vi "check_time_method.vi"(8 "error in (no error)":errorcluster, 9 "Vrijeme od kog se broji":dbl, 10 "Proteklo vrijeme":dbl, 11 "Poslednji vremenski trenutak":dbl) -> (0 "error out":errorcluster, 1 "Status":T1, 2 "Novo proteklo vrijeme":dbl, 3 "Novi vremenski trenutak":dbl)   [LabVIEW 2023]
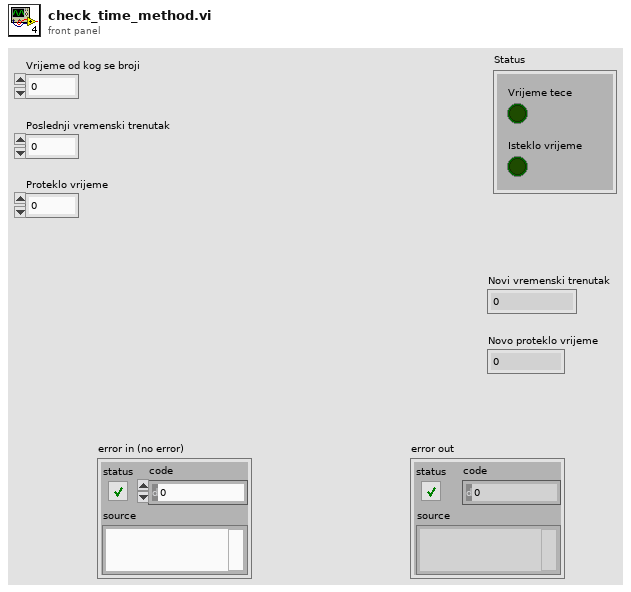
[diagram p1: front panel]
types:
  T1 = cluster{"Vrijeme tece":bool, "Isteklo vrijeme":bool}
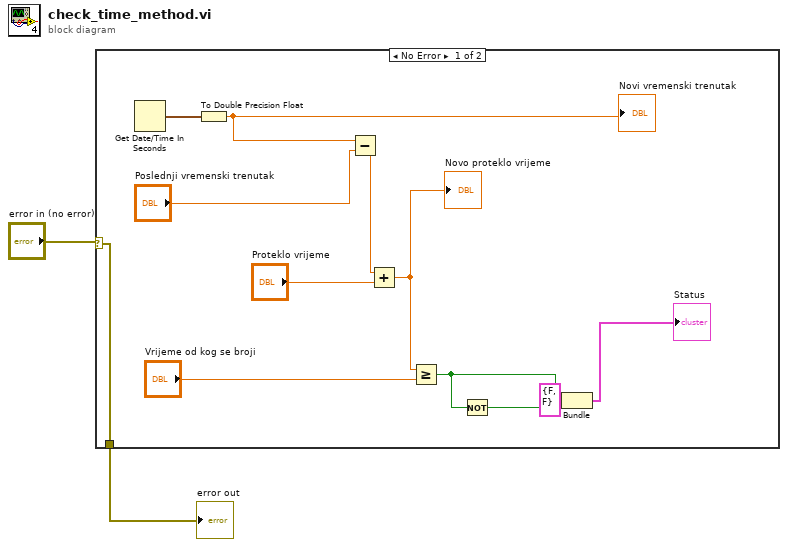
[diagram p0: block diagram]
diagram:
  n1 = case shown="No Error" "error in (no error)" {
    selector: "error in (no error)" -> [w14 w15]
    tunnel: [w14 w15] -> w1
    frame No Error {
      n2 = Get Date/Time In Seconds() -> (seconds since 1Jan1904=w13:timestamp)
      n3 = To Double Precision Float(number=w13) -> (double precision float=w7:dbl)
      "Novi vremenski trenutak" <- w7
      n4 = Subtract(x=w7, y="Poslednji vremenski trenutak") -> (x-y=w11:dbl)
      n5 = Add(x=w11, y="Proteklo vrijeme") -> (x+y=w8:dbl)
      "Novo proteklo vrijeme" <- w8
      n6 = Greater Or Equal?(x=w8, y="Vrijeme od kog se broji") -> (x >= y?=w3:bool)
      n7 = Not(x=w3) -> (.not. x?=w4:bool)
      n8 = Bundle(cluster=cluster{bool, bool} {FALSE, FALSE}, w3, w4) -> (→"Status":cluster{bool, bool})
    }
    frame Error {
    }
  }
  "error out" <- w1
